vi "Initialize Channel Editor State.vi"(8 "error in (no error)":errorcluster, 10 "Module Connection Information":T1[](array[typedef]), 11 "Routing Channel Ref in":T8 format="%.0x") -> (0 "error out":errorcluster, 2 "Channel Editor State":T3, 3 "Routing Channel Ref out":T8 format="%.0x")   [LabVIEW 2020, in "Routing and Faulting System Explorer.lvlib"]
uses:
  Routing and Faulting System Explorer.lvlib
  <vilib>/NI VeriStand/Custom Device API/Custom Device Item Ref.ctl
  Channel Editor State.ctl
  Possible Connections.ctl
  Shared/Routing and Faulting Hardware API/Types/Possible Connections for Endpoint.ctl
  Shared/Alias Mapping.ctl
  Shared/Alias Endpoint.ctl
  Alias Map by Module.ctl
  Scripting/Types/Module Information.ctl
  Shared/Routing and Faulting Shared.lvlib
  Shared/Routing and Faulting Hardware API/Routing and Faulting Hardware API.lvlib
  <vilib>/NI VeriStand/Custom Device API/Custom Device API.lvlib
  Scripting/Routing and Faulting Scripting.lvlib
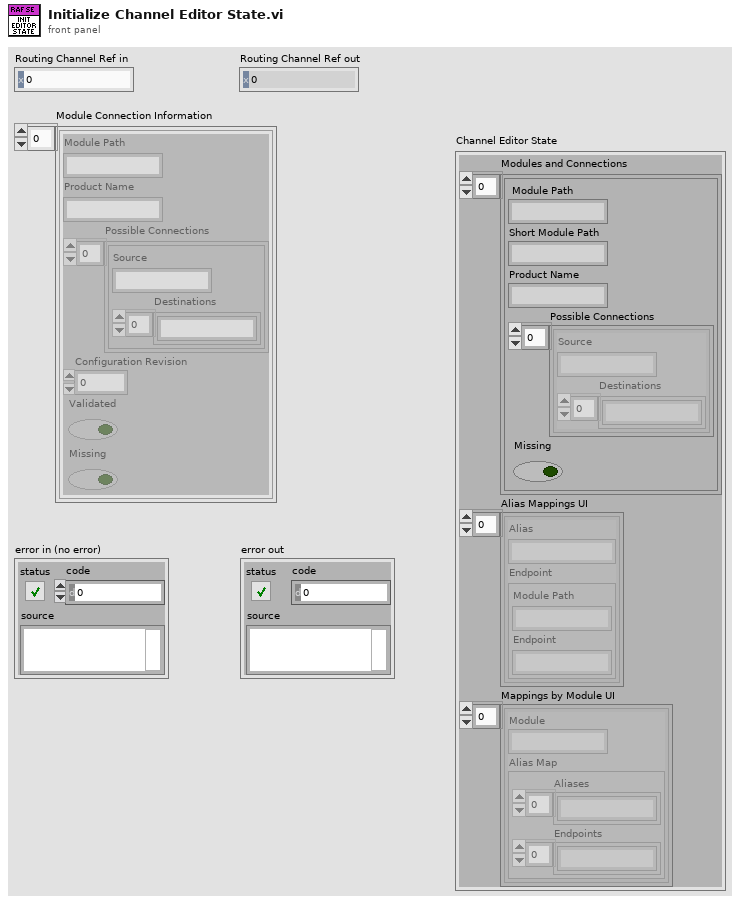
[diagram p1: front panel]
types:
  T1 = typedef "Routing and Faulting Scripting.lvlib/Module Information.ctl" = cluster{"Module Path":string, "Product Name":string, "Possible Connections":T2[], "Configuration Revision":u32, "Validated":bool, "Missing":bool}
  T2 = typedef "Routing and Faulting Hardware API.lvlib/Possible Connections for Endpoint.ctl" = cluster{"Source":string, "Destinations":string[]}
  T3 = typedef "Routing and Faulting System Explorer.lvlib/Channel Editor State.ctl" = cluster{"Modules and Connections":T4[], "Alias Mappings UI":T5[], "Mappings by Module UI":T7[]}
  T4 = typedef "Routing and Faulting System Explorer.lvlib/Possible Connections.ctl" = cluster{" Module Path":string, "Short Module Path":string, "Product Name":string, "Possible Connections":T2[], "Missing":bool}
  T5 = typedef "Routing and Faulting Shared.lvlib/Alias Mapping.ctl" = cluster{"Alias":string, "Endpoint":T6}
  T6 = typedef "Routing and Faulting Shared.lvlib/Alias Endpoint.ctl" = cluster{"Module Path":string, "Endpoint":string}
  T7 = typedef "Routing and Faulting System Explorer.lvlib/Alias Map by Module.ctl" = cluster{"Module":string, "Alias Map":cluster{"Aliases":string[], "Endpoints":string[]}}
  T8 = typedef "Custom Device API.lvlib/Custom Device Item Ref.ctl" = u64
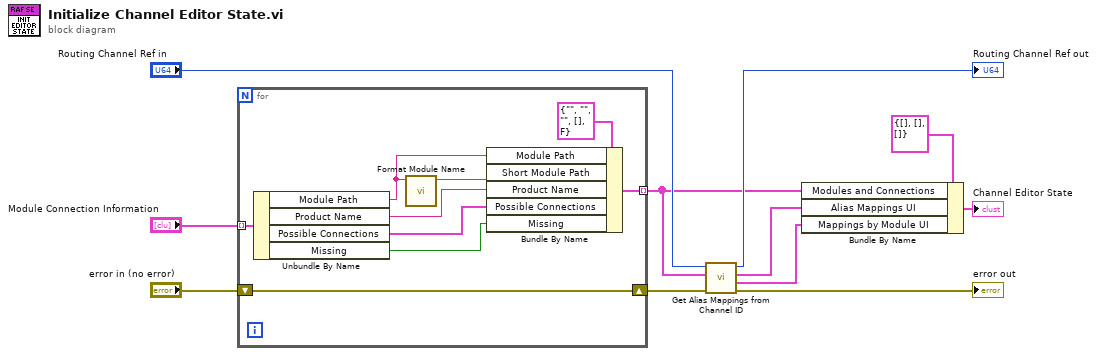
[diagram p0: block diagram]
diagram:
  n1 = for {
    shift-right: [w13] -> w1
    shift-left: "error in (no error)" -> [w13]
    tunnel: [w20] -> w3 mode=indexing
    tunnel: "Module Connection Information" -> [w17] mode=indexing
    n2 = Unbundle By Name(w17) -> ("Module Path"=w16:string, "Product Name"=w15:string, "Possible Connections"=w14:T2[], "Missing"=w12:bool)
    n3 = call "Format Module Name.vi"("Module Path"=w16) -> ("Formatted Module Path"=w19:string)  [unwired: 10 in]
    n4 = Bundle By Name(cluster=T4 {" Module Path"="", "Short Module Path"="", "Product Name"="", "Possible Connections"=[], "Missing"=FALSE} ("Item"), "Module Path"=w16, "Short Module Path"=w19, "Product Name"=w15, "Possible Connections"=w14, "Missing"=w12) -> (w20:T4)
  }
  n5 = call "Get Alias Mappings from Channel ID.vi"("error in (no error)"=w1, "Modules and Connections"=w3, "Routing Channel Ref in"="Routing Channel Ref in") -> ("error out"=→"error out":errorcluster, "Mappings by Module UI"=w6:T7[], "Alias Mappings UI"=w9:T5[], "Routing Channel Ref out"=→"Routing Channel Ref out":T8)  [unwired: 5 in]
  n6 = Bundle By Name(cluster=T3 {"Modules and Connections"=[], "Alias Mappings UI"=[], "Mappings by Module UI"=[]} ("Channel Editor State"), "Modules and Connections"=w3, "Alias Mappings UI"=w9, "Mappings by Module UI"=w6) -> (→"Channel Editor State":T3)
